vi "AlliGator Save FLI Dataset to HDF5 File v3 (VDM).vi"(5 "Compression (T)":bool=TRUE, 6 "Gate Names (Gate)":string[](array[string]), 7 "Software + Version":string, 8 "Error In":errorcluster, 9 "Dataset Information":T2={"Single Dataset Path"=path "", "Dataset ID in Series (1)"=1, "# Datasets in Series (1)"=1, "Dataset Timestamp (s)"=0.0, "Additional Metadata"="", "DAQ Parameters"={"# Pixel X"=0, "# Pixel Y"=0, "# Gates"=0, "# Datasets"=0, "Gate Image Exposure"=0.0, "Macrotime Gate Separation"=0.0, "Nanotime Gate Separation"=0.0, "Gate Width"=0.0, "Laser Period"=0.0, "SYNC Period"=0.0, "Gate Image Integration"=0.0}, "Dataset Data Description"="", "X Bin"=0, "Y Bin"=0}, 10 "Channel 2 Gate Image Array":T1[](array[typedef]), 11 "Channel 1 Gate Image Array":T1[](array[typedef])) -> (0 "Error Out":errorcluster, 3 "File Path out":path, 4 "Time (s)":dbl)   [LabVIEW 2021, in "AlliGator HDF5.lvlib"]
doc: "Save gate images (single- or dual-channel) and dataset information to HDF5 file."
uses:
  AlliGator HDF5.lvlib
  <vilib>/vision/Image Controls.llb/IMAQ Image.ctl
  Files/AlliGator Saved Dataset Information.ctl
  Phasor/Phasor Fluorescence Lifetime Parameters v3.ctl
  <vilib>/addons/h5labview2/file/H5F.lvlib
  Time/Time.lvlib
  Error/Error.lvlib
  Files/AlliGator Files.lvlib
  Phasor/Phasor.lvlib
panel:
  # "see the AlliGator License on the block diagram (Ctrl+E or Window:Show Block Diagram)"
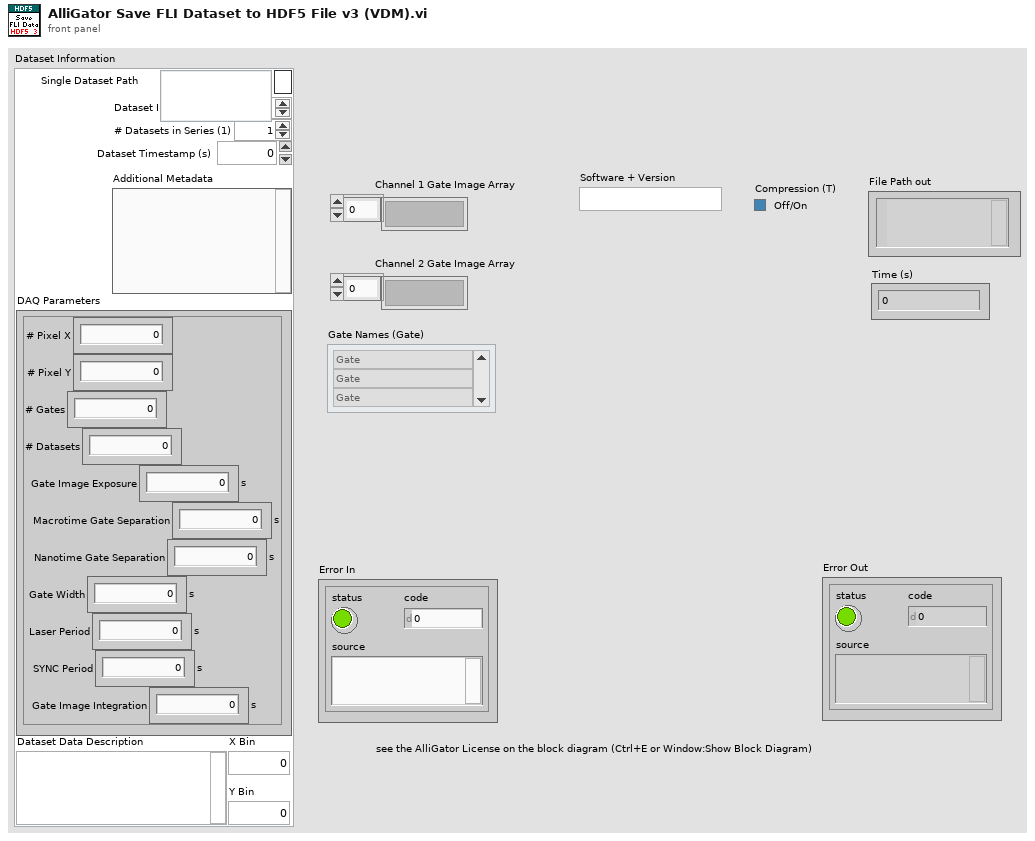
[diagram p1: front panel]
types:
  T1 = typedef "IMAQ Image.ctl" = refnum<image>
  T2 = typedef "AlliGator Files.lvlib/AlliGator Saved Dataset Information.ctl" = cluster{"Single Dataset Path":path, "Dataset ID in Series (1)":i32, "# Datasets in Series (1)":i32, "Dataset Timestamp (s)":dbl, "Additional Metadata":string, "DAQ Parameters":T3, "Dataset Data Description":string, "X Bin":i32, "Y Bin":i32}
  T3 = typedef "Phasor.lvlib/Phasor Fluorescence Lifetime Parameters v3.ctl" = cluster{"# Pixel X":i32, "# Pixel Y":i32, "# Gates":i32, "# Datasets":i32, "Gate Image Exposure":dbl[unit], "Macrotime Gate Separation":dbl[unit], "Nanotime Gate Separation":dbl[unit], "Gate Width":dbl[unit], "Laser Period":dbl[unit], "SYNC Period":dbl[unit], "Gate Image Integration":dbl[unit]}
  T4 = typedef "hid_t.ctl" = i64
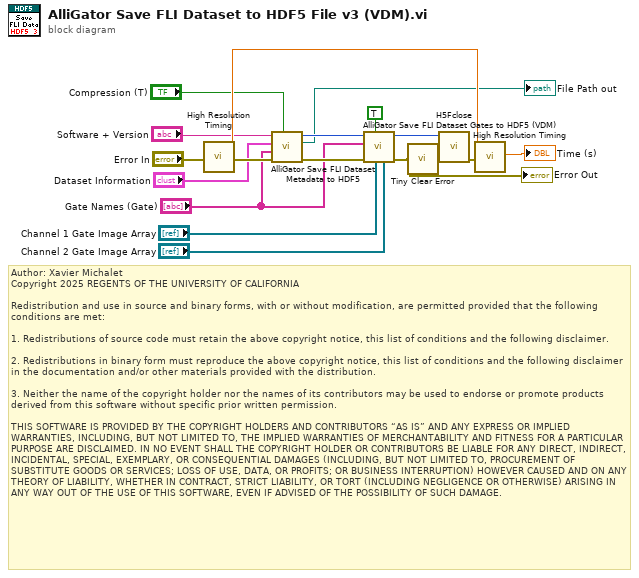
[diagram p0: block diagram]
diagram:
  # "Author: Xavier Michalet\nCopyright 2025 REGENTS OF THE UNIVERSITY OF CALIFORNIA\n\nRedistribution and use in source and binary forms, with or without modification, are permitted provided that the following conditions are met:\n\n1. Redistributions of source code must retain the above copyright notice, this list of conditions and the following disclaimer.\n\n2. Redistributions in binary form must reproduce the above copyright notice, this list of conditions and the following disclaimer in the documentation and/or other materials provided with the distribution.\n\n3. Neither the name of the copyright holder nor the names of its contributors may be used to endorse or promote products derived from this software without specific prior written permission.\n\nTHIS SOFTWARE IS PROVIDED BY THE COPYRIGHT HOLDERS AND CONTRIBUTORS “AS IS” AND ANY EXPRESS OR IMPLIED WARRANTIES, INCLUDING, BUT NOT LIMITED TO, THE IMPLIED WARRANTIES OF MERCHANTABILITY AND FITNESS FOR A PARTICULAR PURPOSE ARE DISCLAIMED. IN NO EVENT SHALL THE COPYRIGHT HOLDER OR CONTRIBUTORS BE LIABLE FOR ANY DIRECT, INDIRECT, INCIDENTAL, SPECIAL, EXEMPLARY, OR CONSEQUENTIAL DAMAGES (INCLUDING, BUT NOT LIMITED TO, PROCUREMENT OF SUBSTITUTE GOODS OR SERVICES; LOSS OF USE, DATA, OR PROFITS; OR BUSINESS INTERRUPTION) HOWEVER CAUSED AND ON ANY THEORY OF LIABILITY, WHETHER IN CONTRACT, STRICT LIABILITY, OR TORT (INCLUDING NEGLIGENCE OR OTHERWISE) ARISING IN ANY WAY OUT OF THE USE OF THIS SOFTWARE, EVEN IF ADVISED OF THE POSSIBILITY OF SUCH DAMAGE."
  n1 = call "High Resolution Timing.vi"("Error In"="Error In") -> ("elapsed (relative) seconds"=w15:dbl, "Error Out"=w16:errorcluster)  [unwired: 16 in, 1 out]
  n2 = call "AlliGator Save FLI Dataset Metadata to HDF5.vi"("Compression"="Compression (T)", "error in (no error)"=w16, "Gate Names"="Gate Names (Gate)", "Dataset Information"="Dataset Information", "Software + Version"="Software + Version") -> ("error out"=w7:errorcluster, "File Path out"=→"File Path out":path, "HDF5 File ref out"=w3:T4)  [unwired: 4 in]
  n3 = call "AlliGator Save FLI Dataset Gates to HDF5 (VDM).vi"("Channel 2 Gate Image Array"="Channel 2 Gate Image Array", "Channel 1 Gate Image Array"="Channel 1 Gate Image Array", "replace?"=TRUE, "error in (no error)"=w7, "Gate Names"="Gate Names (Gate)", "HDF5 File ref in"=w3) -> ("error out"=w12:errorcluster, "HDF5 File ref out"=w10:T4)  [unwired: 4 in]
  "Error Out" <- w12
  n4 = call "Tiny Clear Error.vi"("Error In"=w12) -> ("no Error Out"=w13:errorcluster)  [unwired: 8 in]
  n5 = call <vilib>:"H5Fclose.vi"("error in (no error)"=w13, "ref"=w10) -> ("error out"=w18:errorcluster)  [unwired: 9 in]
  n6 = call "High Resolution Timing.vi"("relative seconds (NaN)"=w15, "Error In"=w18) -> ("elapsed (relative) seconds"=→"Time (s)":dbl)  [unwired: 15 in, 2 out]
